vi "Lockin_Amplifier_diag.vi"(0 "Reference signal (dialog if empty)":path=path "D:/#Meresek/Malaria/Malaria_measurement_program/Labview/Lock_in_Amplifier/tesztsor/timetrace_46.txt", 1 "Sample Number":i32=100000, 2 "DC(V)":dbl, 3 "Cutoff Frequency":dbl=500.0, 4 "dt":dbl=0.0002, 5 "Window (s)":dbl=3.0, 6 "Continous Lock-in":bool, 7 "Resolution":dbl=0.0001, 8 "averaging time":dbl=1.0 format="%0.2p", 9 "Error In":errorcluster, 11 "Second":bool, 12 "Sampling Freq":dbl=5000.0, 14 "tolerance (Deviation)":dbl=3.0) -> (13 "Error Out":errorcluster, 15 "dLD_RMS":dbl, 16 "LD_RMS":dbl, 17 "Signal Spectrum":cluster{"f0":dbl, "df":dbl, "magnitude":dbl[]}[](graph), 18 "LockIN R (cont/disc)":waveform(dbl)[](graph), 19 "LD(cont/disc)":T1, 20 "Lock-in R (Vrms)":cluster{dbl[], "Result":dbl[]}(graph), 21 "Lock-in Theta":cluster{dbl[], "Result":dbl[]}(graph), 23 "Time Domain Signal":cluster{"xi used":dbl[], "yi":dbl[]}[](graph), 24 "Phase average":dbl format="%0.2f", 25 "Phase  deviation":dbl format="%0.2f", 27 "Integral":cluster{dbl[], dbl[]}[](graph))   [LabVIEW 2013]
uses:
  <vilib>/Utility/file.llb/Read From Spreadsheet File (DBL).vi
  <vilib>/gmath/NI_Gmath.lvlib
  <vilib>/Analysis/NI_AALBase.lvlib
panel:
  out "Averaging window":dbl
  in  "Tab Control":T2(tab)
  out "Reference signal / PLL Signal":cluster{"all rows":dbl[], "all rows":dbl[]}[](graph)
  out "Reference Spectrum":cluster{"f0":dbl, "df":dbl, "magnitude":dbl[]}(graph)
  out "Synthetized Spectrum":cluster{"f0":dbl, "df":dbl, "magnitude":dbl[]}(graph)
  in  "t0_ref":dbl
  in  "t0_LD":dbl=0.0001
  out "LD Spectrum (Vrms)":cluster{"f0":dbl, "df":dbl, "magnitude":dbl[]}(graph)
  out "LD Signal":cluster{"all rows":dbl[], "all rows":dbl[]}[](graph)
  out "Tolerance Level":dbl
  out "average":dbl
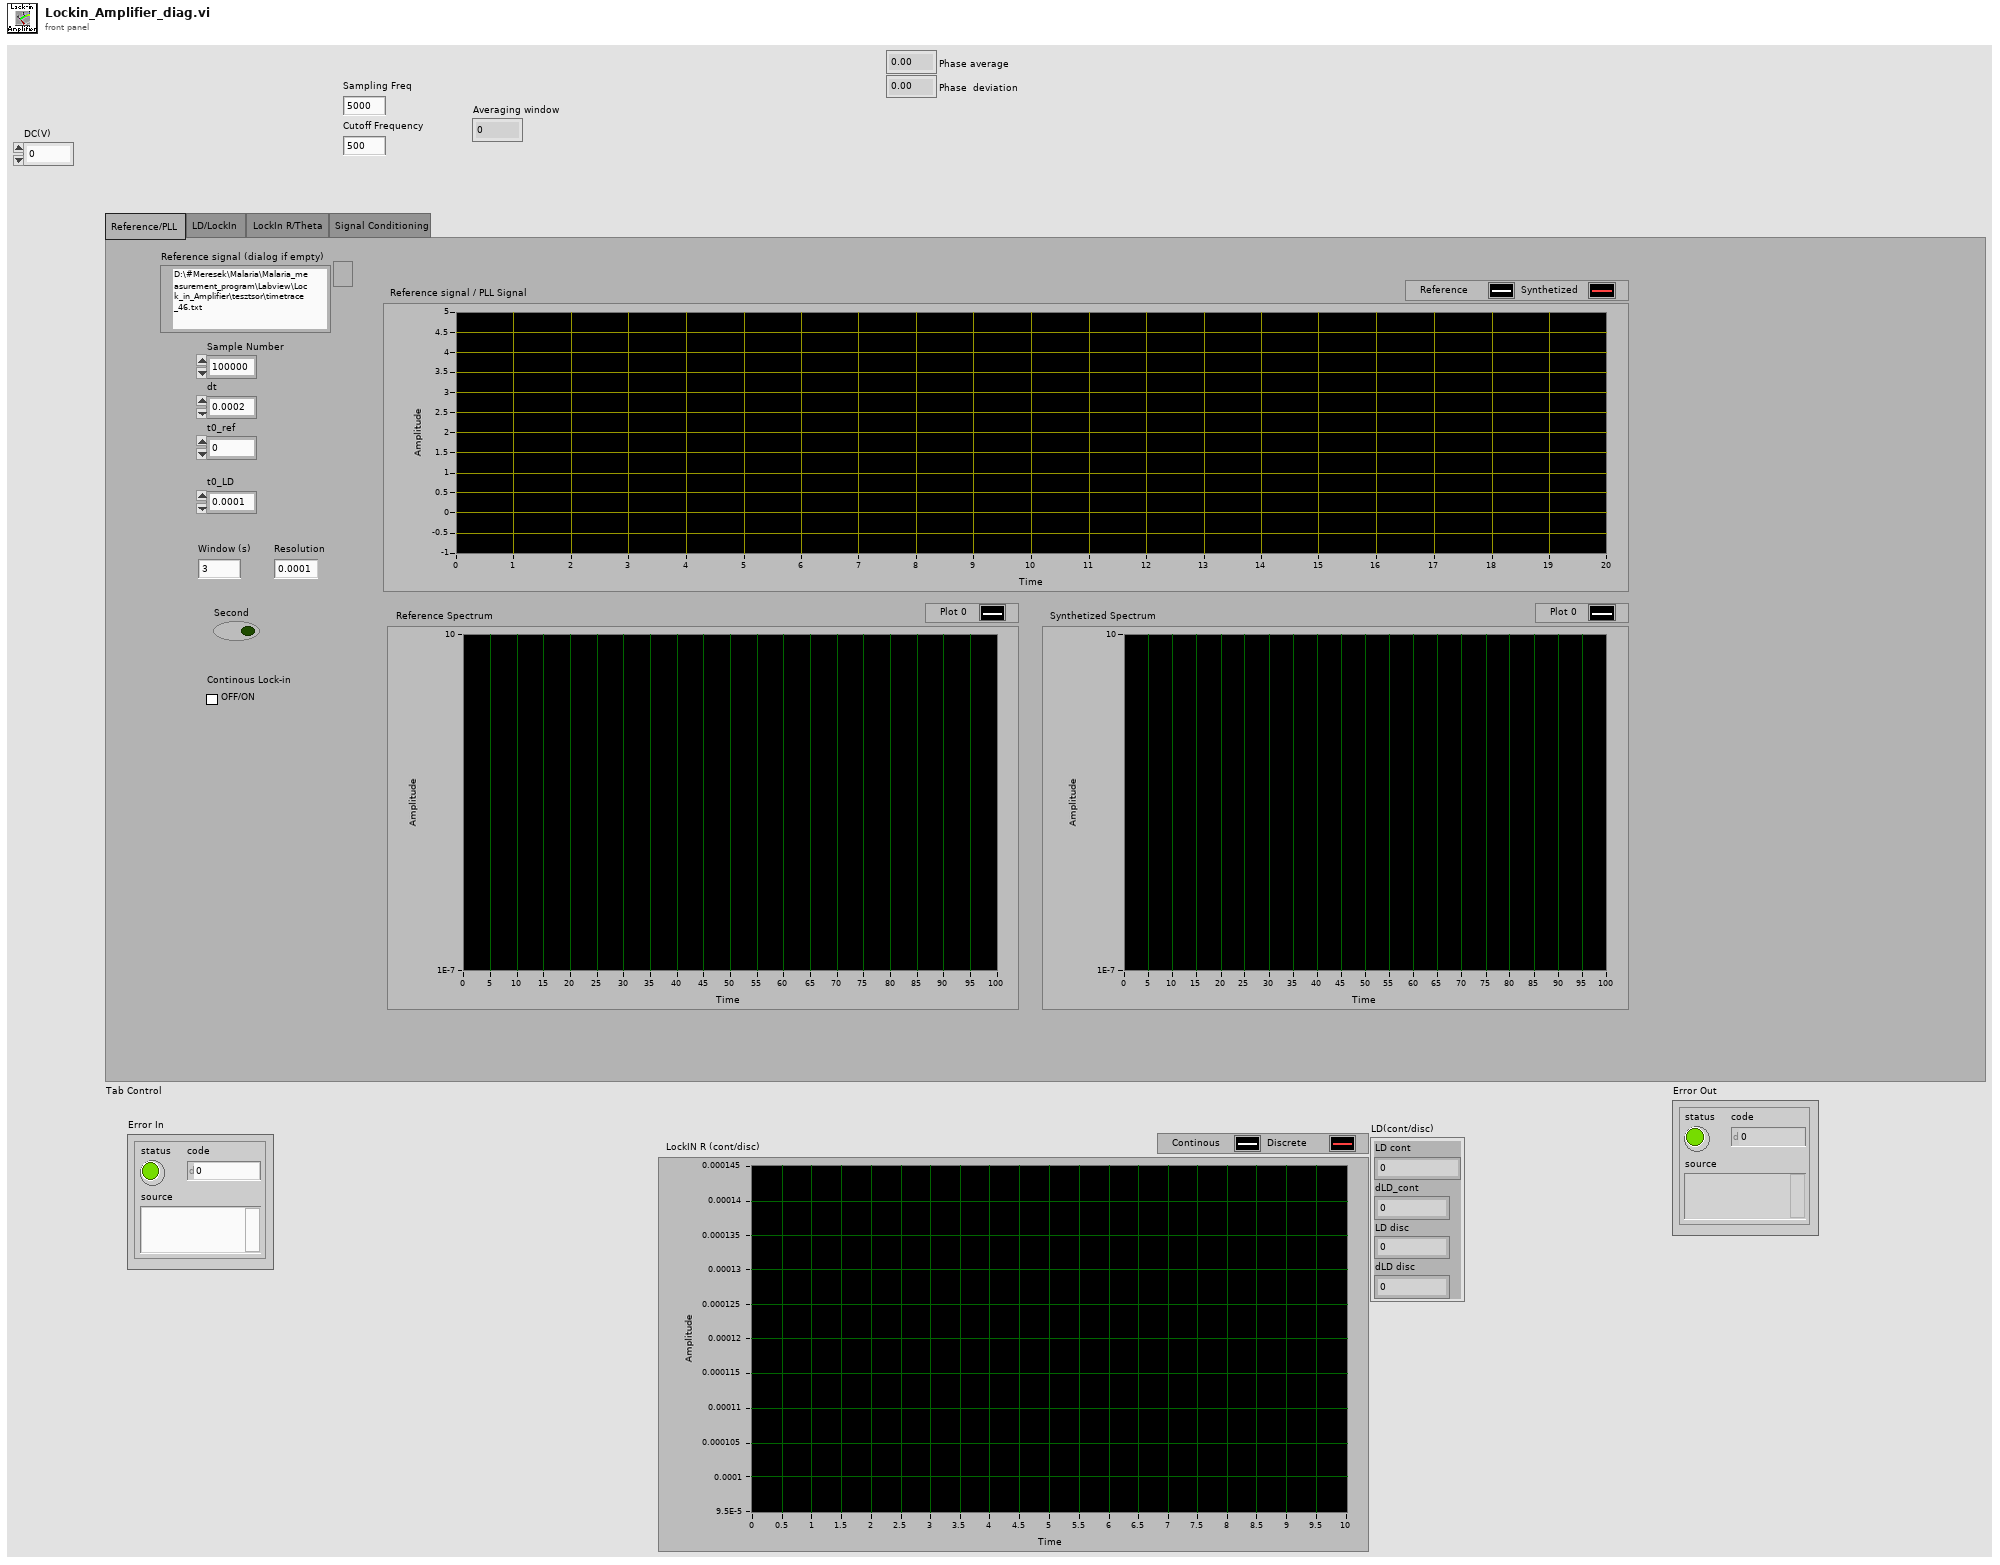
[diagram p1: front panel]
types:
  T1 = cluster{"LD cont":dbl, "dLD_cont":dbl, "LD disc":dbl, "dLD disc":dbl}
  T2 = enum32{"Reference/PLL", "LD/LockIn", "LockIn R/Theta", "Signal Conditioning"}
  T3 = cluster{"mean":dbl, "standard deviation":dbl, "mean":dbl, "standard deviation":dbl}
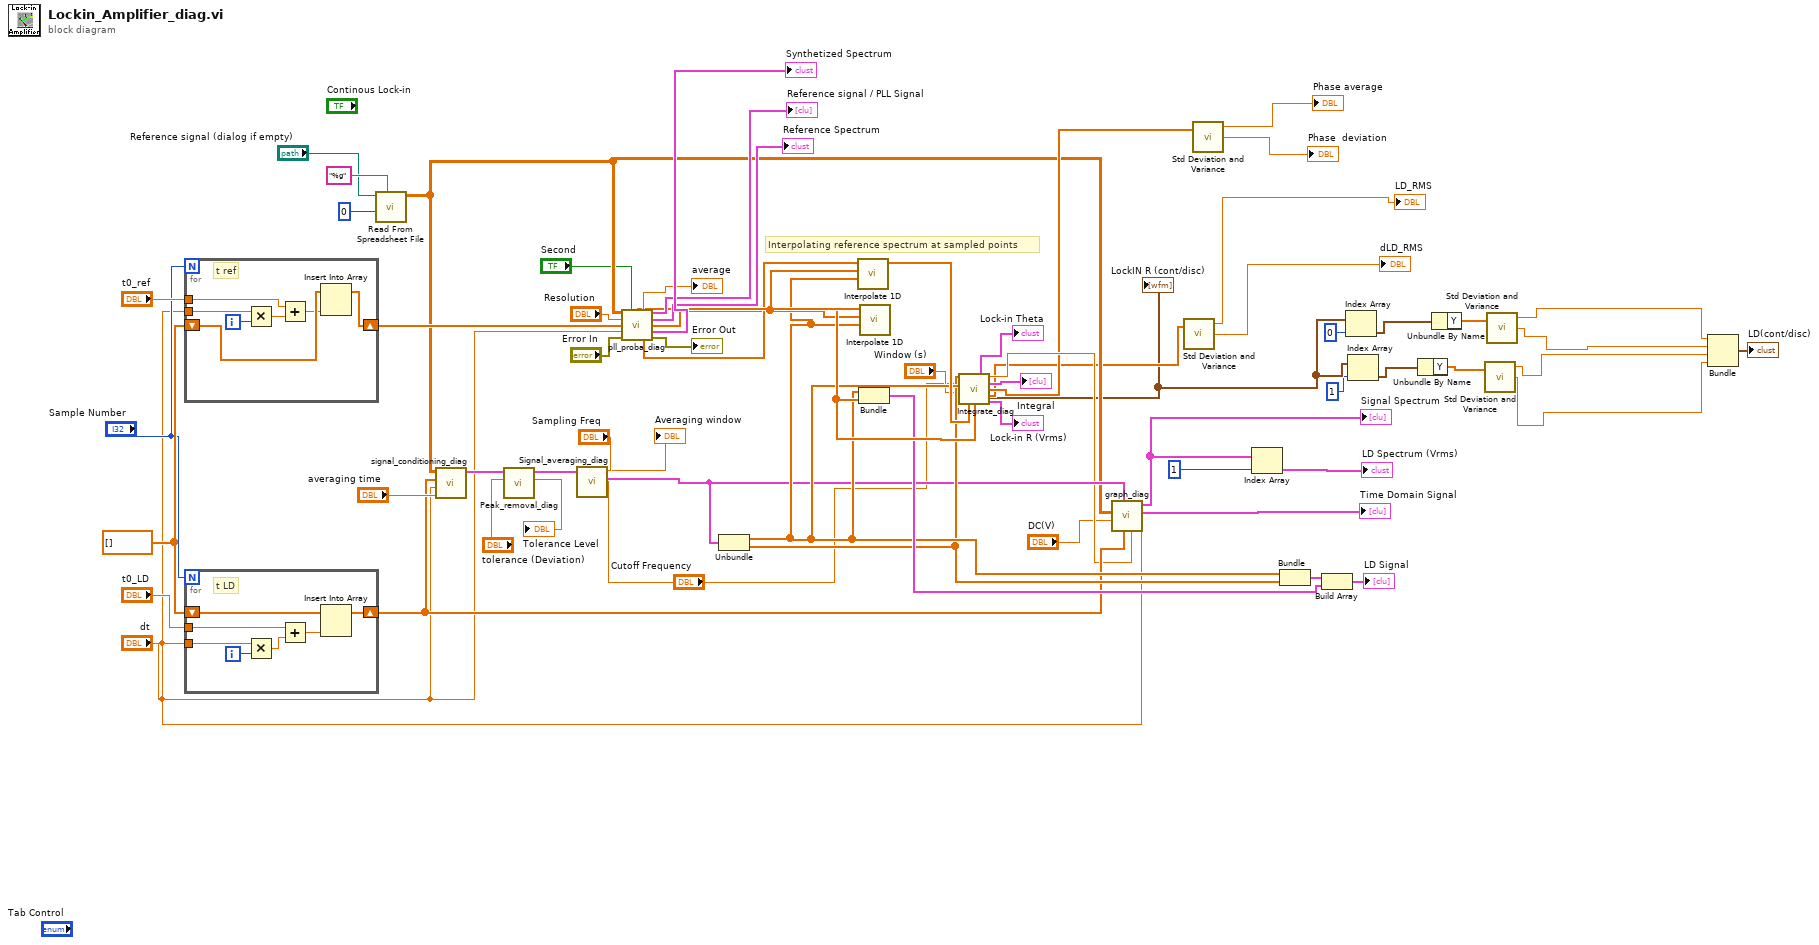
[diagram p0: block diagram]
diagram:
  w39 = dbl[] []
  # "Interpolating reference spectrum at sampled points"
  n1 = for {
    N: "Sample Number" -> [_]
    shift-right: [w72] -> w40
    shift-left: w39 -> [w71]
    tunnel: "dt" -> [w70]
    tunnel: "t0_ref" -> [w69]
    i -> [w73]
    # "t ref"
    n2 = Multiply(x=w70, y=w73) -> (x*y=w68:dbl)
    n3 = Add(x=w69, y=w68) -> (x+y=w67:dbl)
    n4 = Insert Into Array(array=w71, new element=w67) -> (w72:dbl[])  [unwired: 1 in]
  }
  n5 = for {
    N: "Sample Number" -> [_]
    shift-right: [w79] -> w36
    shift-left: w39 -> [w78]
    tunnel: "dt" -> [w77]
    tunnel: "t0_LD" -> [w76]
    i -> [w80]
    # "t LD"
    n6 = Multiply(x=w77, y=w80) -> (x*y=w75:dbl)
    n7 = Add(x=w76, y=w75) -> (x+y=w74:dbl)
    n8 = Insert Into Array(array=w78, new element=w74) -> (w79:dbl[])  [unwired: 1 in]
  }
  n9 = call-poly <vilib>:"Read From Spreadsheet File.vi"("format (%.3f)"="%g" ("format (%.6f)"), "start of read offset (chars.:0)"=0, "file path (dialog if empty)"="Reference signal (dialog if empty)") -> ("all rows"=w17:dbl[][])  [unwired: 4 in, 4 out]
  n10 = call "signal_conditioning_diag.vi"("averaging time"="averaging time", "dt"="dt", "t_LD"=w36, "all rows"=w17) -> ("Offset removed"=w42:cluster{"xi used":dbl[], "yi":dbl[]})  [unwired: 6 in, 1 out]
  n11 = call "Peak_removal_diag.vi"("tolerance (Deviation)"="tolerance (Deviation)", "Offset removed"=w42) -> ("Tolerance Level"=→"Tolerance Level":dbl, "XY Graph"=w34:cluster{"xi used":dbl[], "yi":dbl[]})  [unwired: 8 in]
  n12 = call "Signal_averaging_diag.vi"("Pike removed"=w34, "Cutoff Frequency"="Cutoff Frequency", "Sampling Freq"="Sampling Freq") -> ("Averaged"=w33:cluster{"xi used":dbl[], "yi":dbl[]}, "Averaging window"=→"Averaging window":dbl)  [unwired: 7 in]
  n13 = call "pll_proba_diag.vi"("all rows"=w17, "Second"="Second", "Resolution"="Resolution", "t_ref"=w40, "dt"="dt", "Error In"="Error In") -> ("average"=→"average":dbl, "XY Graph"=→"Reference signal / PLL Signal":cluster{"all rows":dbl[], "all rows":dbl[]}[], "Waveform Graph"=→"Reference Spectrum":cluster{"f0":dbl, "df":dbl, "magnitude":dbl[]}, "time"=w50:dbl[], "Waveform Graph 2"=→"Synthetized Spectrum":cluster{"f0":dbl, "df":dbl, "magnitude":dbl[]}, "PLL_sine"=w54:dbl[], "PLL_cosine"=w51:dbl[], "Error Out"=→"Error Out":errorcluster)  [unwired: 2 in]
  n14 = Unbundle(w33) -> ("xi used"=w46:dbl[], "yi"=w45:dbl[])
  n15 = call <vilib>:"Interpolate 1D.vi"("xi"=w46, "X"=w50, "Y"=w51) -> ("yi"=w49:dbl[])  [unwired: 6 in, 2 out]
  n16 = call <vilib>:"Interpolate 1D.vi"("xi"=w46, "X"=w50, "Y"=w54) -> ("yi"=w53:dbl[])  [unwired: 6 in, 2 out]
  n17 = Bundle("xi used"=w46, "yi"=w53) -> (w52:cluster{"xi used":dbl[], "yi":dbl[]})  [unwired: 1 in]
  n18 = call "Integrate_diag.vi"("Processed LD values"=w45, "Processed LD time values"=w46, "Cutoff Frequency"="Cutoff Frequency", "Window (s)"="Window (s)", "Ref Sine"=w49, "Ref Cosine"=w53) -> ("Lockin Theta"=→"Lock-in Theta":cluster{dbl[], "Result":dbl[]}, "Numeric"=w28:dbl, "Lock in X,Y,R (Vrms) time"=→"Integral":cluster{dbl[], "Result":dbl[]}[], "LockIn Theta Array"=w23:dbl[], "LockIn R (Vrms) array"=w13:dbl[], "LockIN R (cont/disc)"=w12:waveform(dbl)[], "LockIn R (Vrms)"=→"Lock-in R (Vrms)":cluster{dbl[], "Result":dbl[]})  [unwired: 3 in]
  "LockIN R (cont/disc)" <- w12
  n19 = call "graph_diag.vi"(4:"dt"=w28, "Array in"=w36, "Averaged"=w33, "DC(V)"="DC(V)", "LD Timetrace in"=w17, 11:"dt"="dt") -> ("Time Domain Signal"=→"Time Domain Signal":cluster{"xi used":dbl[], "yi":dbl[]}[], "Spectra"=w26:cluster{"f0":dbl, "df":dbl, "magnitude":dbl[]}[])  [unwired: 4 in]
  "Signal Spectrum" <- w26
  n20 = call <vilib>:"Std Deviation and Variance.vi"("X"=w13) -> ("mean"=→"LD_RMS":dbl, "standard deviation"=→"dLD_RMS":dbl)  [unwired: 1 in, 1 out]
  n21 = call <vilib>:"Std Deviation and Variance.vi"("X"=w23) -> ("mean"=→"Phase average":dbl, "standard deviation"=→"Phase  deviation":dbl)  [unwired: 1 in, 1 out]
  n22 = Index Array(array=w26, index=1) -> (element=→"LD Spectrum (Vrms)":cluster{"f0":dbl, "df":dbl, "magnitude":dbl[]})
  n23 = Bundle("xi used"=w46, "yi"=w45) -> (w55:cluster{"xi used":dbl[], "yi":dbl[]})  [unwired: 1 in]
  n24 = Build Array(w55, w52) -> (→"LD Signal":cluster{"xi used":dbl[], "yi":dbl[]}[])
  n25 = Index Array(array=w12, index=0) -> (element=w9:waveform(dbl))
  n26 = Index Array(array=w12, index=1) -> (element=w8:waveform(dbl))
  n27 = Unbundle By Name(w8) -> ("Y"=w6:dbl[])
  n28 = Unbundle By Name(w9) -> ("Y"=w7:dbl[])
  n29 = call <vilib>:"Std Deviation and Variance.vi"("X"=w6) -> ("mean"=w3:dbl, "standard deviation"=w2:dbl)  [unwired: 1 in, 1 out]
  n30 = call <vilib>:"Std Deviation and Variance.vi"("X"=w7) -> ("mean"=w5:dbl, "standard deviation"=w4:dbl)  [unwired: 1 in, 1 out]
  n31 = Bundle("mean"=w5, "standard deviation"=w4, "mean"=w3, "standard deviation"=w2) -> (→"LD(cont/disc)":T3)  [unwired: 1 in]
